vi "Time since T0 high performance.vi"(4 "error in (no error)":errorcluster, 6 "T0 ticks value":u64, 7 "Variant (for data flow only)":variant) -> (0 "error out":errorcluster, 2 "Time elapsed (ms)":dbl format="%.2f", 3 "current ticks":u64)   [LabVIEW 2012]
doc: "This vi measures the time in milliseconds since T0. The variant input is unused. It is provided to establish dataflow with .vi's that do not have error outputs."
uses:
  kernel32.dll
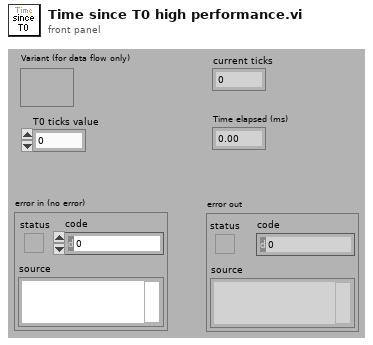
[diagram p1: front panel]
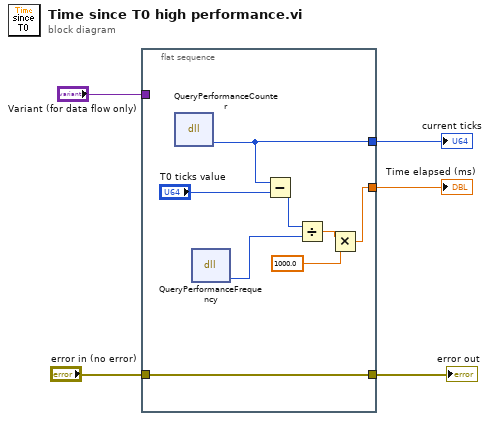
[diagram p0: block diagram]
diagram:
  n1 = flat-sequence {
    tunnel: [w6] -> w5
    tunnel: [w12] -> w4
    tunnel: [w11] -> w3
    tunnel: "error in (no error)" -> [w12]
    tunnel: "Variant (for data flow only)" -> [_]
    frame #0 {
      n2 = dll-call lib="kernel32.dll" fn="QueryPerformanceCounter"() -> ("pPerformanceCount"=w11:u64)  [unwired: 5 in, 2 out]
      n3 = dll-call lib="kernel32.dll" fn="QueryPerformanceFrequency"() -> ("pTicksPerSecond"=w9:u64)  [unwired: 5 in, 2 out]
      n4 = Subtract(x=w11, y="T0 ticks value") -> (x-y=w10:u64)
      n5 = Divide(x=w10, y=w9) -> (x/y=w8:dbl)
      n6 = Multiply(x=w8, y=1000.0) -> (x*y=w6:dbl)
    }
  }
  "Time elapsed (ms)" <- w5
  "error out" <- w4
  "current ticks" <- w3
